vi "mod_Selective Resample profile to requested sampling rate.vi"(0 "doppler filter output":cdb[](array[numeric]), 7 "profile length (samples)":i32=1000, 9 "interpolation factor":i32=1, 11 "error in (no error)":errorcluster, 13 "reset? (T)":bool=TRUE) -> (4 "fading profile":cdb[](array[numeric]), 15 "error out":errorcluster)   [LabVIEW 2020, in "niDMT.lvlib"]
uses:
  <vilib>/addons/Modulation/niDMT.lvlib
  <vilib>/addons/Modulation/Analog/support/mod_Generate Integer Interpolation Filter.vi
  <vilib>/addons/Modulation/niAMT.lvlib
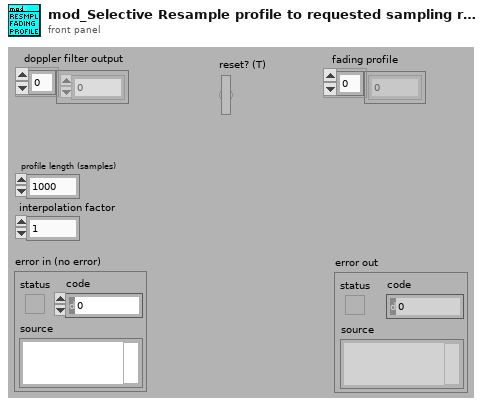
[diagram p1: front panel]
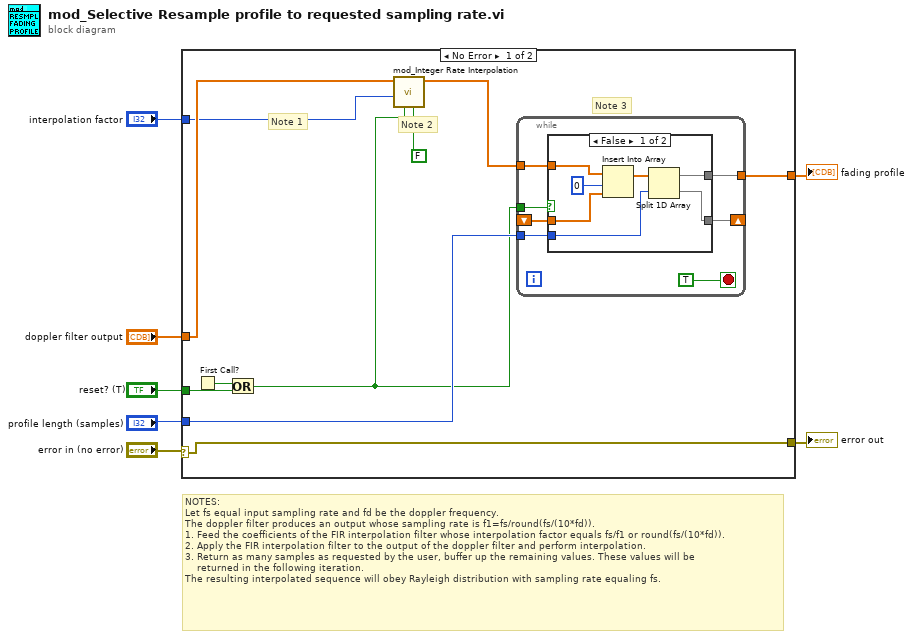
[diagram p0: block diagram]
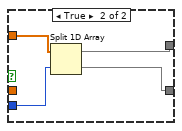
[diagram p2: hidden frame]
diagram:
  # "NOTES:\nLet fs equal input sampling rate and fd be the doppler frequency.\nThe doppler filter produces an output whose sampling rate is f1=fs/round(fs/(10*fd)).\n1. Feed the coefficients of the FIR interpolation filter whose interpolation factor equals fs/f1 or round(fs/(10*fd)).\n2. Apply the FIR interpolation filter to the output of the doppler filter and perform interpolation.\n3. Return as many samples as requested by the user, buffer up the remaining values. These values will be \n    returned in the following iteration.\nThe resulting interpolated sequence will obey Rayleigh distribution with sampling rate equaling fs."
  n1 = case shown="No Error" "error in (no error)" {
    selector: "error in (no error)" -> [w10 w36]
    tunnel: "interpolation factor" -> [w12 _]
    tunnel: "reset? (T)" -> [w17 _]
    tunnel: "profile length (samples)" -> [w15 _]
    tunnel: "doppler filter output" -> [w13 _]
    tunnel: [w10 w36] -> w2
    tunnel: [w14 _] -> w1
    frame No Error {
      # "Note 3"
      # "Note 2"
      # "Note 1"
      n2 = First Call?() -> (First Call?: T/F=w16:bool)
      n3 = Or(x=w16, y=w17) -> (x .or. y?=w8:bool)
      n4 = call <vilib>:"mod_Integer Rate Interpolation.vi"("flush buffers? (F)"=FALSE ("flush? (F)"), "reset? (T)"=w8, "interpolation factor"=w12, "input[]"=w13) -> ("output[]"=w11:cdb[])  [unwired: 7 out]
      n5 = while {
        tunnel: w8 -> [w23]
        tunnel: w11 -> [w22]
        tunnel: w15 -> [w21]
        shift-right: [w20] -> _
        shift-left: _ -> [w19]
        tunnel: [w18] -> w14
        stop <- TRUE stop-if-true
        n6 = case shown="False" w23 {
          tunnel: w22 -> [w31 w35]
          tunnel: w21 -> [w27 w34]
          tunnel: [w26 w33] -> w20
          tunnel: w19 -> [w29 _]
          tunnel: [w25 w32] -> w18
          frame False {
            n7 = Insert Into Array(array=w31, index=0, new element=w29) -> (w28:cdb[])
            n8 = Split 1D Array(array=w28, index=w27) -> (first subarray=w25:cdb[], second subarray=w26:cdb[])
          }
          frame True {
            n9 = Split 1D Array(array=w35, index=w34) -> (first subarray=w32:cdb[], second subarray=w33:cdb[])
          }
        }
      }
    }
    frame Error {
    }
  }
  "error out" <- w2
  "fading profile" <- w1
